vi "Module Add and Max.vi"(7 "channel":T1, 10 "self":string caption="self subchannel", 11 "caller":string caption="caller subchannel") -> ()   [LabVIEW 2020]
uses:
  1cd8508f-c559-4445-93fb-4c26ceb1d59b.vi
  7c0fa1f5-a764-4cd0-8de9-1a51003f9f17.vi
  38333639-7e8e-41e1-89a3-0328f237a635.vi
  <extravilib>/ChannelInstances/Event MessengerM-c(str,var)/))Channel.ctl
  <extravilib>/ChannelInstances/Event MessengerM-c(str,var).lvlib
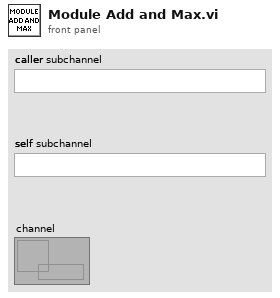
[diagram p1: front panel]
types:
  T1 = typedef "Event MessengerM-c(str,var).lvlib/))Channel.ctl" = refnum<queue>
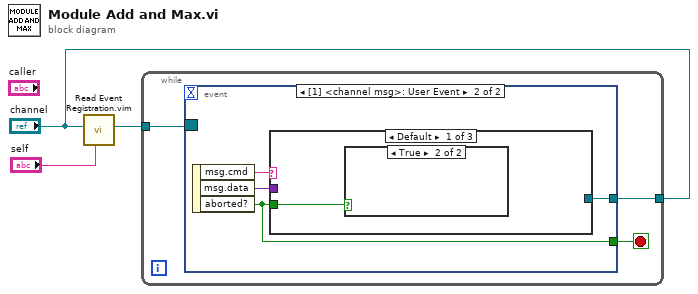
[diagram p0: block diagram]
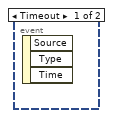
[diagram p2: hidden frame]
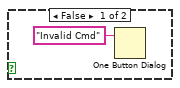
[diagram p3: hidden frame]
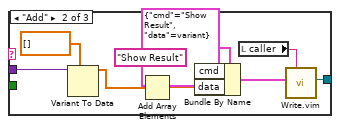
[diagram p4: hidden frame]
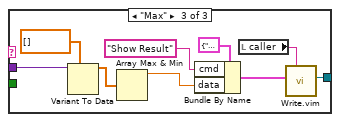
[diagram p5: hidden frame]
diagram:
  n1 = call "Read Event Registration.vim"("subchannel"="self", "channel"="channel") -> ("event registration refnum"=w3:refnum<event-registration>)  [unwired: 9 in]
  n2 = while {
    tunnel: w3 -> [w6]
    tunnel: "channel" -> [w4]
    stop <- w5 stop-if-true
    n3 = event shown="[1] <channel msg>: User Event" {
      selector: w6 -> [_ _]
      dyn-events: _ -> [_ _]
      timeout: _ -> [_ _]
      tunnel: [_ w7] -> w5
      tunnel: [_ w8] -> w4
      event Timeout {
        n4 = event-data() -> ()  [unwired: 1 in, 3 out]
      }
      event User Event {
        n5 = event-data() -> ("msg.cmd"=w10:string, "msg.data"=w9:variant, "aborted?"=w7:bool)  [unwired: 1 in]
        n6 = case shown="Default" w10 {
          tunnel: w9 -> [_ w18 w27]
          tunnel: [_ w14 w23] -> w8
          tunnel: w7 -> [w11 _ _]
          frame Default {
            n7 = case shown="True" w11 {
              frame False {
                n8 = One Button Dialog(message="Invalid Cmd") -> ()  [unwired: 1 in, 1 out]
              }
              frame True {
              }
            }
          }
          frame "Add" {
            n9 = Variant To Data(type=dbl[] [], Variant=w18) -> (data=w16:dbl[])  [unwired: 1 in, 1 out]
            n10 = Add Array Elements(numeric array=w16) -> (sum=w13:dbl)
            n11 = Bundle By Name(cluster=cluster{"cmd":string, "data":variant} {"cmd"="Show Result", "data"=variant}, "cmd"="Show Result", "data"=w13) -> (w21:cluster{"cmd":string, "data":variant})
            n12 = local read "caller"() -> (w15:string)
            n13 = call "Write.vim"("subchannel"=w15, "element"=w21) -> ("channel"=w14:T1)  [unwired: 8 in, 1 out]
          }
          frame "Max" {
            n14 = Variant To Data(type=dbl[] [], Variant=w27) -> (data=w25:dbl[])  [unwired: 1 in, 1 out]
            n15 = Array Max & Min(array=w25) -> (max value=w22:dbl)  [unwired: 3 out]
            n16 = Bundle By Name(cluster=cluster{"cmd":string, "data":variant} {"cmd"="Show Result", "data"=variant}, "cmd"="Show Result", "data"=w22) -> (w30:cluster{"cmd":string, "data":variant})
            n17 = local read "caller"() -> (w24:string)
            n18 = call "Write.vim"("subchannel"=w24, "element"=w30) -> ("channel"=w23:T1)  [unwired: 8 in, 1 out]
          }
        }
      }
    }
  }
